vi "開啟圖片(1D).vi"(8 "error In":errorcluster, 10 "Image Name":string="Source", 11 "影像數量":i32=1) -> (0 "error out":errorcluster, 1 "ImageOutNameArray":string[](array[string]), 2 "ImagePathNumber":i32, 3 "ImagePath":path[](array[path]))   [LabVIEW 2015]
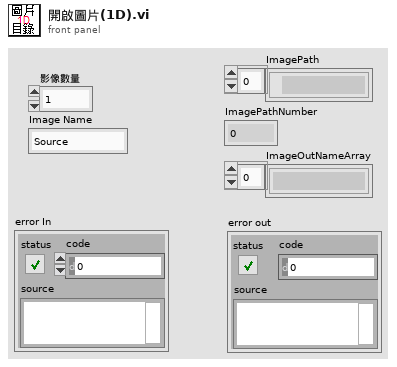
[diagram p1: front panel]
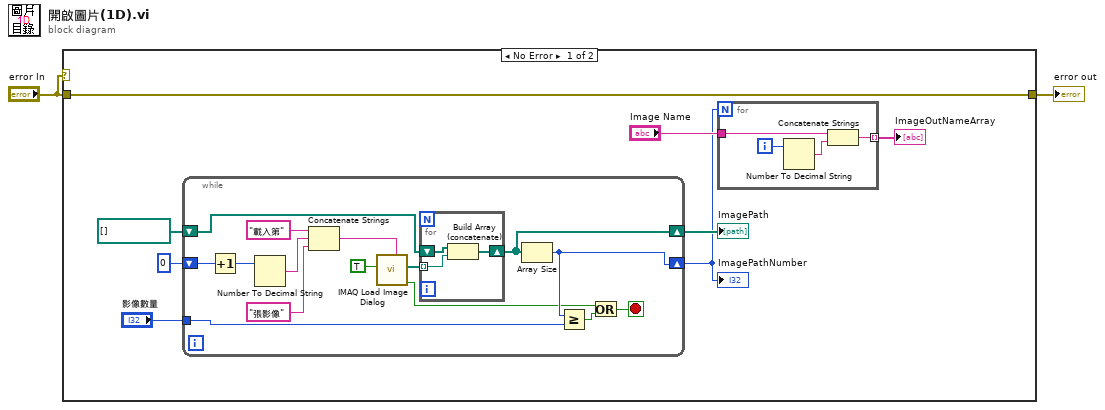
[diagram p0: block diagram]
diagram:
  n1 = case shown="No Error" "error In" {
    tunnel: [w6 w33] -> w2
    tunnel: "error In" -> [w6 w33]
    frame No Error {
      n2 = while {
        tunnel: "影像數量" -> [w26]
        shift-right: [w29] -> w7
        shift-left: path[] [] -> [w25]
        shift-right: [w24] -> w4
        shift-left: 0 -> [w23]
        stop <- w16 stop-if-true
        n3 = Increment(x=w23) -> (x+1=w22:i32)
        n4 = Number To Decimal String(number=w22) -> (decimal integer string=w19:string)  [unwired: 1 in]
        n5 = Concatenate Strings("載入第", w19, "張影像") -> (w18:string)
        n6 = call "IMAQ Load Image Dialog"("Button Label"=w18, "Multiple Files? (No)"=TRUE) -> ("Cancelled?"=w17:bool, "Paths"=w27:path[])  [unwired: 7 in, 1 out]
        n7 = for {
          tunnel: w27 -> [w31] mode=indexing
          shift-right: [w30] -> w29
          shift-left: w25 -> [w32]
          n8 = Build Array (concatenate)(w32, w31) -> (w30:path[])
        }
        n9 = Array Size(array=w29) -> (size(s)=w24:i32)
        n10 = Greater Or Equal?(x=w24, y=w26) -> (x >= y?=w15:bool)
        n11 = Or(x=w17, y=w15) -> (x .or. y?=w16:bool)
      }
      "ImagePath" <- w7
      "ImagePathNumber" <- w4
      n12 = for {
        N: w4 -> [_]
        tunnel: "Image Name" -> [w13]
        tunnel: [w11] -> w3 mode=indexing
        i -> [w14]
        n13 = Number To Decimal String(number=w14) -> (decimal integer string=w12:string)  [unwired: 1 in]
        n14 = Concatenate Strings(w13, w12) -> (w11:string)
      }
      "ImageOutNameArray" <- w3
    }
    frame Error {
    }
  }
  "error out" <- w2
